vi "Average temperature.vi"() -> ()   [LabVIEW 2014]
doc: "This VI is the solution to an exercise in the LabVIEW Core I course.\n\nIt is used to demonstrate While loops and waveform charts. This VI simulates a temperature reading once every 500 ms and plots the data in a strip chart."
panel:
  out "Temperature History":dbl(graph)
  in  "Power":bool=TRUE
  # "ON\n\nOFF"
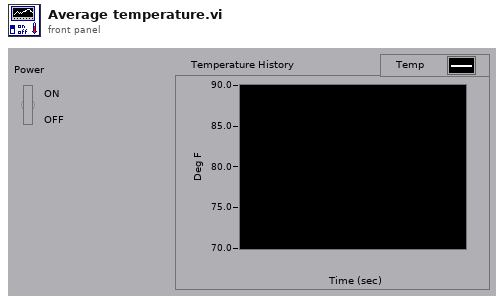
[diagram p1: front panel]
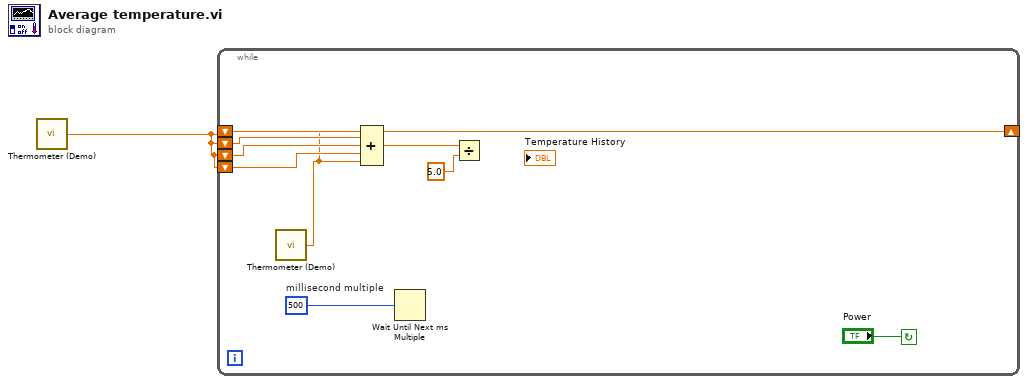
[diagram p0: block diagram]
diagram:
  n1 = call "Thermometer (Demo).vi"() -> ("Temperature"=w1:dbl)  [unwired: 1 in]
  n2 = while {
    shift-right: [w2] -> _
    shift-left: w1 -> [w8]
    shift-left: w1 -> [w7]
    shift-left: w1 -> [w5]
    shift-left: w1 -> [w6]
    stop <- "Power" continue-if-true
    w9 = u32 500  # millisecond multiple
    n3 = call "Thermometer (Demo).vi"() -> ("Temperature"=w2:dbl)  [unwired: 1 in]
    n4 = Compound Arithmetic op=ADD(w8, w7, w6, w5, w2) -> (w4:dbl)
    n5 = Wait Until Next ms Multiple(millisecond multiple=w9) -> ()  [unwired: 1 out]
    n6 = Divide(x=w4, y=5.0 ("x/y")) -> ()  [unwired: 1 out]
  }
